vi "Convert_data_to_string_MOA.vi"(0 "Data":T1, 5 "Wavelenght [nm]":dbl format="%#_13g", 7 "Min/Max Voltage [V]":dbl format="%#_13g", 9 "X Shift [V]":dbl format="%#_13g", 11 "Y Shift [V]":dbl format="%#_13g") -> (4 "spreadsheet string":string)   [LabVIEW 2018]
doc: "This VI enables to convert the measurements data to a string.\n\nInput:\n(1) Data: the data cluster.\nThis cluster contains the Threshold power [W], the number of seconds from the beginning and the measurement time stamp.\n\nOutput:\n(1) Spreadsheet string - the string which contains the measurement data"
uses:
  Data_MOA.ctl
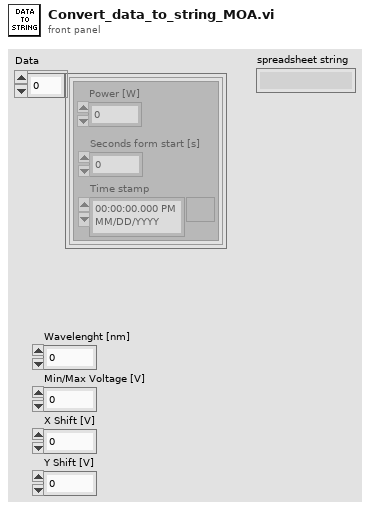
[diagram p1: front panel]
types:
  T1 = typedef "Data_MOA.ctl" = cluster{cluster{"Power [W]":dbl, "Seconds form start [s]":dbl, "Time stamp":timestamp}}[]
  T2 = cluster{"Power [W]":dbl, "Seconds form start [s]":dbl, "Time stamp":timestamp}
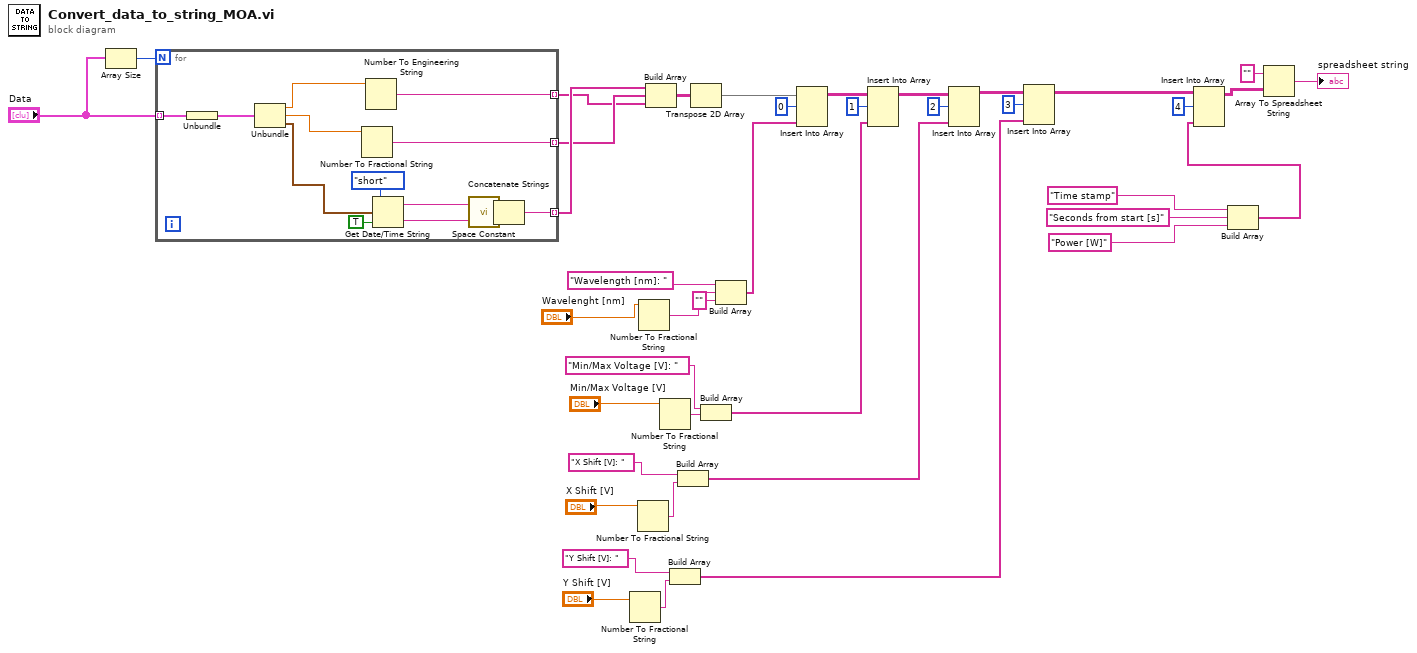
[diagram p0: block diagram]
diagram:
  n1 = Array Size(array="Data") -> (size(s)=w35:i32)
  n2 = for {
    N: w35 -> [_]
    tunnel: "Data" -> [w49] mode=indexing
    tunnel: [w43] -> w8 mode=indexing
    tunnel: [w44] -> w39 mode=indexing
    tunnel: [w45] -> w40 mode=indexing
    n3 = Unbundle(w49) -> (w53:T2)
    n4 = Unbundle(w53) -> ("Power [W]"=w50:dbl, "Seconds form start [s]"=w42:dbl, "Time stamp"=w41:timestamp)
    n5 = Number To Fractional String(number=w42) -> (F-format string=w44:string)  [unwired: 3 in]
    n6 = Number To Engineering String(4:w50) -> (0:w43:string)  [unwired: 3 in]
    n7 = Get Date/Time String(date format (0)=enum16{"short", "long", "abbreviated"}."short", seconds (now)=w41, want seconds? (F)=TRUE) -> (date string=w48:string, time string=w46:string)
    n8 = call <vilib>:"Space Constant.vi"() -> ("String"=w47:string)
    n9 = Concatenate Strings(w48, w47, w46) -> (w45:string)
  }
  n10 = Number To Fractional String(number="Y Shift [V]") -> (F-format string=w11:string)  [unwired: 3 in]
  n11 = Number To Fractional String(number="X Shift [V]") -> (F-format string=w17:string)  [unwired: 3 in]
  n12 = Number To Fractional String(number="Wavelenght [nm]") -> (F-format string=w29:string)  [unwired: 3 in]
  n13 = Build Array(w40, w39, w8) -> (w36:string[][])
  n14 = Number To Fractional String(number="Min/Max Voltage [V]") -> (F-format string=w20:string)  [unwired: 3 in]
  n15 = Build Array("Y Shift [V]: " ("element"), w11) -> (w14:string[])
  n16 = Build Array("X Shift [V]: " ("element"), w17) -> (w16:string[])
  n17 = Transpose 2D Array(2D array=w36) -> (transposed array=w34:string[][])
  n18 = Build Array("Min/Max Voltage [V]: " ("element"), w20) -> (w21:string[])
  n19 = Build Array("Wavelength [nm]: ", w29, "" ("element")) -> (w32:string[])
  n20 = Insert Into Array(array=w34, index (row)=0, new element=w32) -> (w25:string[][])  [unwired: 1 in]
  n21 = Insert Into Array(array=w25, index (row)=1, new element=w21) -> (w24:string[][])  [unwired: 1 in]
  n22 = Insert Into Array(array=w24, index (row)=2, new element=w16) -> (w23:string[][])  [unwired: 1 in]
  n23 = Insert Into Array(array=w23, index (row)=3, new element=w14) -> (w5:string[][])  [unwired: 1 in]
  n24 = Build Array("Time stamp", "Seconds from start [s]", "Power [W]") -> (w2:string[])
  n25 = Insert Into Array(array=w5, index (row)=4, new element=w2) -> (w4:string[][])  [unwired: 1 in]
  n26 = Array To Spreadsheet String(array=w4, 3:"" ("format string")) -> (spreadsheet string=→"spreadsheet string":string)  [unwired: 1 in]
